vi "Configure Edge Trigger.vi"(0 "device session in":refnum<class "Device Session.lvclass">, 1 "trigger source":u8, 5 "trigger slope":T5, 7 "trigger level (V)":dbl, 9 "hysteresis (%fs)":dbl=0.25, 11 "error in":errorcluster, 12 "instance":enum16{"A", "B"}(ring)) -> (4 "device session out":refnum<class "Device Session.lvclass">, 6 "scaling coefficients":T4[](array[typedef]), 15 "error out":errorcluster)   [LabVIEW 2021, in "Device Session.lvclass"]
doc: "Configures the edge trigger for the selected channel. You can specify the trigger level, hysteresis, and trigger slope.\n\n<B>Input Parameters</B>\n\n<B>device session in</B> is a reference to the Device Session object, which contains a session to each instrument design library used in this sample project. This parameter is obtained from the 'Open Session' VI.\n\n<B>trigger source</B> specifies the channel to monitor for trigger conditions.\n\n<B>trigger slope</B> specifies whether the oscilloscope should trigger on a rising edge or a falling edge.\n\n<B>trigger level (V)</B> specifies the voltage threshold for the trigger.\n\n<B>hysteresis (%fs)</B> specifies in volts the size of the hysteresis window on either side of the specified 'level'. The oscilloscope triggers when the 'trigger source' signal passes through the 'hysteresis level' you specify with this parameter, has the specified 'trigger slope', and passes through the specified 'level'.\n\n<B>instance</B> specifies either instance A or B of the trigger to use.\n\n<B>error in</B> describes error conditions that occur before this node runs. This input provides standard 'error in' functionality.\n\n<B>Output Parameters</B>\n\n<B>device session out</B> passes a reference to the session to the next VI.\n\n<B>error out</B> contains error information. This output provides standard 'error out' functionality."
uses:
  Device Session.lvclass
  <instrlib>/_niInstr/Data Trigger/v1/Shared/Public/Edge Configuration Trigger Slope.ctl
  <instrlib>/_niInstr/Multirecord Acquisition/Interface/v1/Host/Public/Scaling Coefficient.ctl
  Clusts/AllWindowsClust.ctl
  Clusts/ChannelWindowClust.ctl
  Device Session.lvclass/Device Session.ctl
  <vilib>/Utility/error.llb/Error Cluster From Error Code.vi
  <vilib>/rvi/errors/niLvFpgaAdjustHostInterfaceError.vi
  <vilib>/rvi/interface/nirviReadWriteControl/nirviReadWriteControl.xnode
  FPGA Refnum.ctl
  <vilib>/rvi/interface/Simulation/niFpgaSimulationCallBeginRW.vi
  NiFpgaLv.dll
  <instrlib>/_niInstr/Data Trigger/v1/Shared/niInstr Data Trigger v1 Shared.lvlib
  <instrlib>/_niInstr/Multirecord Acquisition/Interface/v1/Host/niInstr Multirecord Acquisition v1 Host.lvclass
panel:
  in  "AllWindows 2":T1
  in  "AllWindows":T3
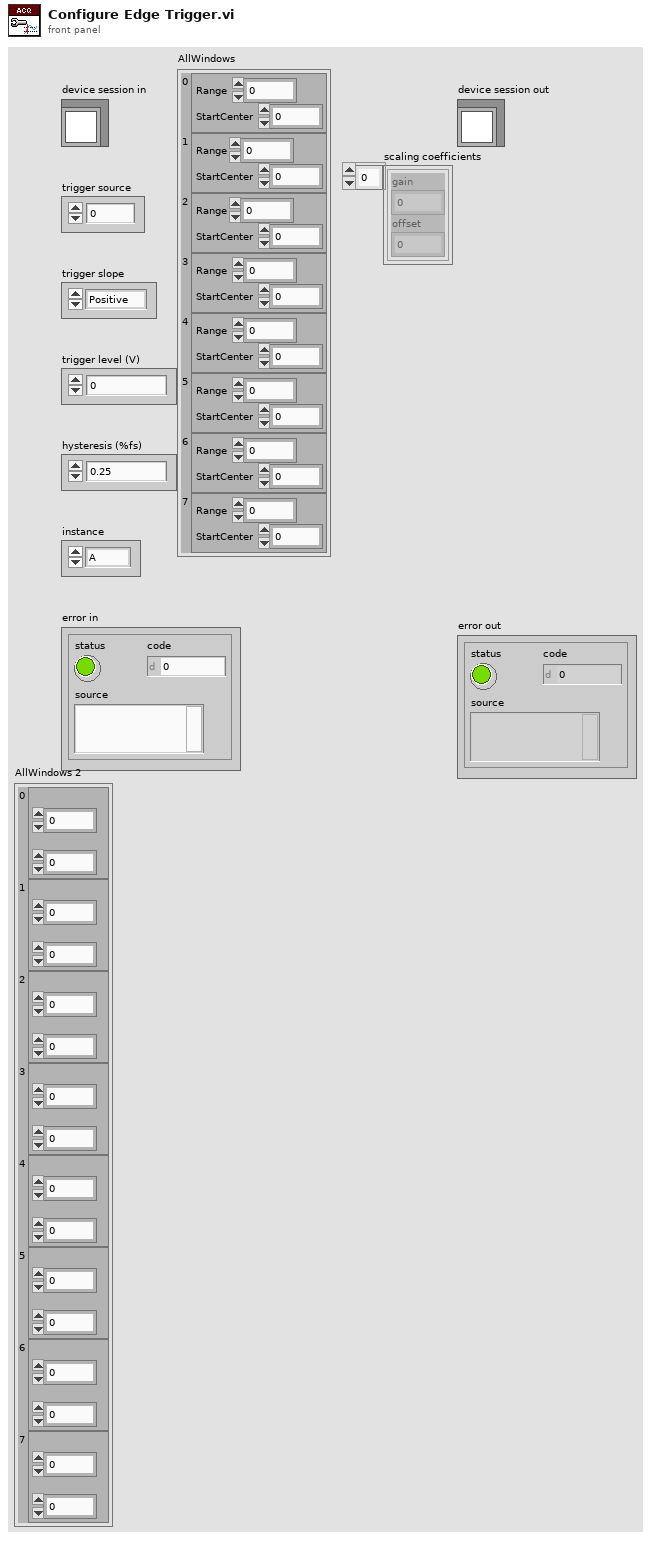
[diagram p1: front panel]
types:
  T1 = typedef "AllWindowsClust.ctl" = cluster{"0":T2, "1":T2, "2":T2, "3":T2, "4":T2, "5":T2, "6":T2, "7":T2}
  T2 = typedef "ChannelWindowClust.ctl" = cluster{"HalfRange":fxp<+/-,18,5>, "StartCenter":fxp<+/-,18,5>}
  T3 = cluster{"0":cluster{"Range":dbl, "StartCenter":dbl}, "1":cluster{"Range":dbl, "StartCenter":dbl}, "2":cluster{"Range":dbl, "StartCenter":dbl}, "3":cluster{"Range":dbl, "StartCenter":dbl}, "4":cluster{"Range":dbl, "StartCenter":dbl}, "5":cluster{"Range":dbl, "StartCenter":dbl}, "6":cluster{"Range":dbl, "StartCenter":dbl}, "7":cluster{"Range":dbl, "StartCenter":dbl}}
  T4 = typedef "niInstr Multirecord Acquisition v1 Host.lvclass/Scaling Coefficient.ctl" = cluster{"gain":dbl, "offset":dbl}
  T5 = typedef "niInstr Data Trigger v1 Shared.lvlib/Edge Configuration Trigger Slope.ctl" = enum8{"Positive", "Negative"}
  T6 = enum16{"Immediate", "A", "B", "OR", "AND", "A THEN B", "B THEN A", "High Resolution"}
  T7 = typedef "Device Session.lvclass/Device Session Object.ctl" = cluster{"fpga reference":T8, "reg bus":refnum<class "niInstr FIFO Register Bus v1 Host.lvclass">, "subsystem map":refnum<class "niInstr Subsystem Map v1 Host.lvclass">, "cal data":refnum<class "niHSAI Cal Data v1 Host.lvclass">, "config":refnum<class "niHSAI Group A Config v1 Host.lvclass">, "acquisition":refnum<class "niInstr Multirecord Acquisition v1 Host.lvclass">, "number of selected acq channels":u8, "selected acq channels":bool[], "number of channels":u32, "configured channels":bool[], "acq configuration":cluster{"number of samples":u64, "number of records":u64, "pretrigger samples":u64}, "actual channel configuration":T9[], "sample clock rate (Hz)":dbl, "scaling coefficients":T4[]}
  T8 = typedef "Device Session.lvclass/FPGA Refnum.ctl" = refnum<k20>
  T9 = typedef "niHSAI Types v1 Host.lvlib/Channel Configuration.ctl" = cluster{"channel":u32, "coupling":T10, "impedance":T11, "bandwidth":T12, "vertical range":dbl, "vertical offset":dbl}
  T10 = typedef "niHSAI Types v1 Host.lvlib/Coupling.ctl" = enum8{"Default", "DC", "AC"}
  T11 = typedef "niHSAI Types v1 Host.lvlib/Impedance.ctl" = enum8{"Default", "1 mega ohm", "50 ohm"}
  T12 = typedef "niHSAI Types v1 Host.lvlib/Bandwidth.ctl" = enum8{"Default", "Full Bandwidth", "Anti-alias Filter", "150 MHz"}
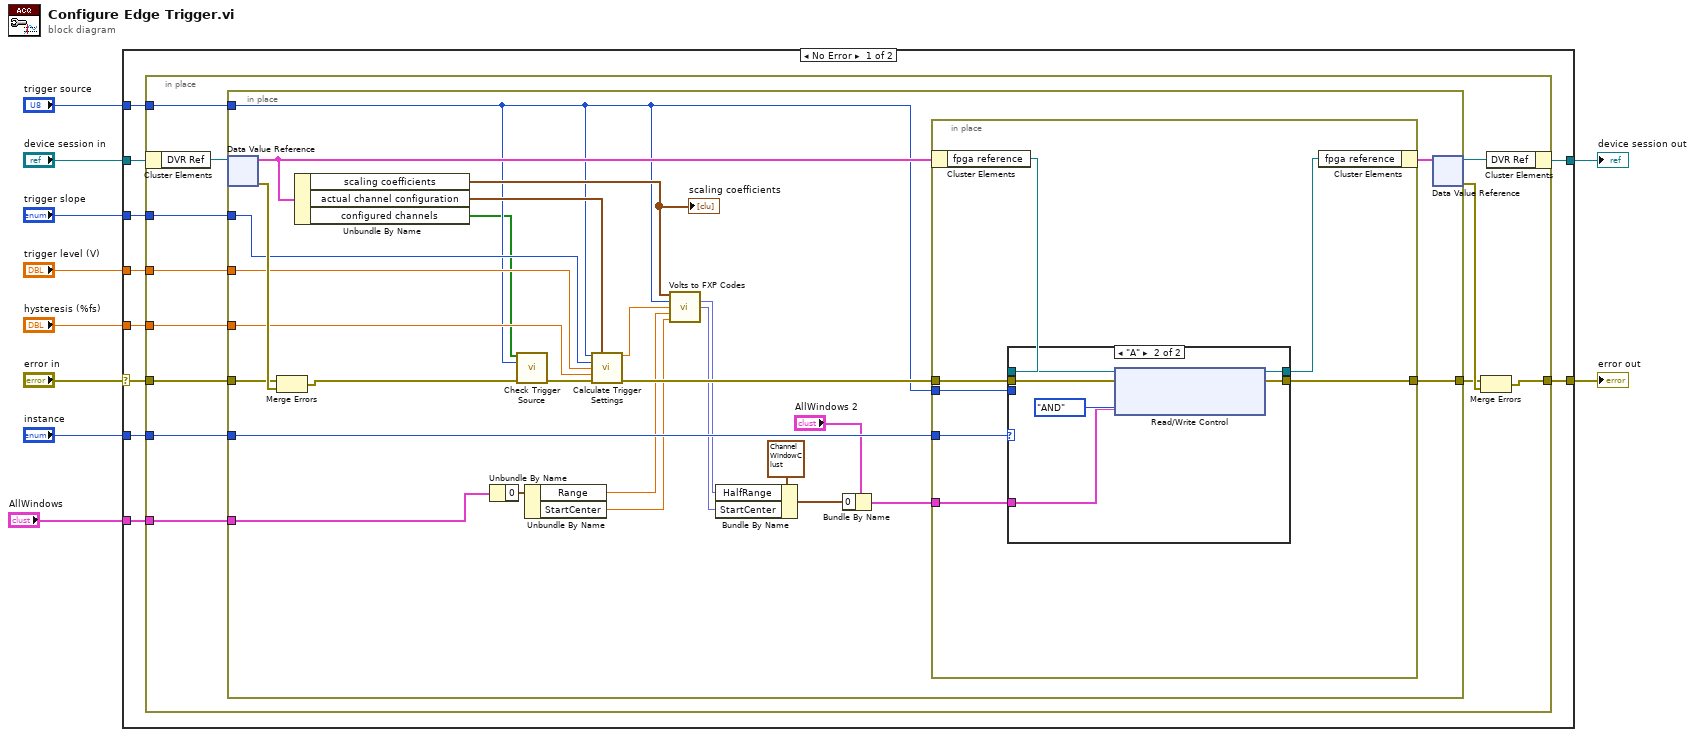
[diagram p0: block diagram]
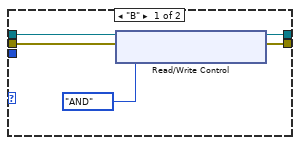
[diagram p2: hidden frame]
diagram:
  n1 = case shown="No Error" "error in" {
    selector: "error in" -> [w20 w79]
    tunnel: "device session in" -> [w13 w78]
    tunnel: [w12 w78] -> w9
    tunnel: [w14 w79] -> w10
    tunnel: "trigger source" -> [w19 _]
    tunnel: "trigger slope" -> [w18 _]
    tunnel: "trigger level (V)" -> [w17 _]
    tunnel: "hysteresis (%fs)" -> [w16 _]
    tunnel: "instance" -> [w15 _]
    tunnel: "AllWindows" -> [w11 _]
    frame No Error {
      n2 = in-place {
        in-place-border: w20 -> [w32]
        in-place-border: w19 -> [w31]
        in-place-border: w18 -> [w30]
        in-place-border: w17 -> [w29]
        in-place-border: w16 -> [w28]
        in-place-border: w15 -> [w26]
        in-place-border: [w24] -> w14
        in-place-border: w11 -> [w21]
        n3 = in-place-cluster #1(w13) -> ("DVR Ref"=w23:refnum<data-value>)
        n4 = in-place {
          in-place-border: w32 -> [w58]
          in-place-border: w31 -> [w44]
          in-place-border: w30 -> [w46]
          in-place-border: w29 -> [w51]
          in-place-border: w28 -> [w50]
          in-place-border: w26 -> [w57]
          in-place-border: [w56] -> w25
          in-place-border: w21 -> [w42]
          n5 = in-place-dvr #2(w23) -> (w48:T7, w59:errorcluster)
          n6 = Merge Errors(w58, w59) -> (w49:errorcluster)
          n7 = Unbundle By Name(w48) -> ("scaling coefficients"=w52:T4[], "actual channel configuration"=w53:T9[], "configured channels"=w43:bool[])
          "scaling coefficients" <- w52
          n8 = Unbundle By Name(w42) -> ("0"=w41:cluster{"Range":dbl, "StartCenter":dbl})
          n9 = call "Check Trigger Source.vi"("configured channels"=w43, "trigger source"=w44, "error in"=w49) -> ("error out"=w55:errorcluster)  [unwired: 12 in]
          n10 = Unbundle By Name(w41) -> ("Range"=w40:dbl, "StartCenter"=w39:dbl)
          n11 = call "Calculate Trigger Settings.vi"("trigger source"=w44, "actual channel configuration"=w53, "trigger slope"=w46, "level (V)"=w51, "hysteresis (%fs)"=w50, "error in"=w55) -> ("high level (V)"=w45:dbl, "error out"=w54:errorcluster)  [unwired: 7 in, 1 out]
          n12 = call "Volts to FXP Codes.vi"("scaling coefficients"=w52, "channel index"=w44, "level (V)"=w45, "Range (V)"=w40, "Center (V)"=w39) -> ("range (fxp)"=w37:fxp<+/-,18,1>, "Center (fxp)"=w36:fxp<+/-,18,1>)  [unwired: 8 in, 1 out]
          n13 = Bundle By Name(cluster=T2 {"HalfRange"=0.0, "StartCenter"=0.0} ("0"), "HalfRange"=w37, "StartCenter"=w36) -> (w34:T2)
          n14 = Bundle By Name(cluster="AllWindows 2", "0"=w34) -> (w33:T1)
          n15 = in-place {
            in-place-border: w57 -> [w66]
            in-place-border: [w65] -> w56
            in-place-border: w54 -> [w64]
            in-place-border: w44 -> [w63]
            in-place-border: w33 -> [w60]
            n16 = in-place-cluster #3(w48) -> ("fpga reference"=w62:T8)
            n17 = case shown="\"A\"" w66 {
              tunnel: w64 -> [w71 w77]
              tunnel: w63 -> [_ _]
              tunnel: [w70 w76] -> w65
              tunnel: w62 -> [w68 w73]
              tunnel: [w67 w74] -> w61
              tunnel: w60 -> [_ w72]
              frame "B" {
                n18 = xnode "Read/Write Control"("FPGA VI Reference In"=w68, "error in"=w71, "trigger.combination type"=T6."AND" ("trigger.combination.type")) -> ("FPGA VI Reference Out"=w67:T8, "error out"=w70:errorcluster)
              }
              frame "A" {
                n19 = xnode "Read/Write Control"("FPGA VI Reference In"=w73, "error in"=w77, "trigger.combination type"=T6."AND" ("trigger.combination.type"), "UserTrig"=w72) -> ("FPGA VI Reference Out"=w74:T8, "error out"=w76:errorcluster)
              }
            }
            n20 = in-place-cluster #3("fpga reference"=w61) -> (w47:T7)
          }
          n21 = in-place-dvr #2(w47) -> (w22:refnum<data-value>, w27:errorcluster)
        }
        n22 = Merge Errors(w25, w27) -> (w24:errorcluster)
        n23 = in-place-cluster #1("DVR Ref"=w22) -> (w12:refnum<class "Device Session.lvclass">)
      }
    }
    frame Error {
    }
  }
  "error out" <- w10
  "device session out" <- w9
